vi "Stop Motor.vi"(9 "Current voltage":dbl, 10 "Desired voltage":dbl, 11 "Refnum in":refnum<k21>) -> ()   [LabVIEW 2018]
uses:
  <vilib>/Analysis/NI_AALBase.lvlib
  <vilib>/Analysis/1siggen.llb/Ramp Pattern by Samples.vi
  Samples per channle (Generation) - Global Variable.vi
  <vilib>/DAQmx/write.llb/DAQmx Write (Analog 1D DBL 1Chan NSamp).vi
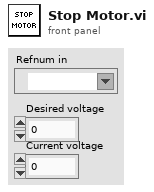
[diagram p1: front panel]
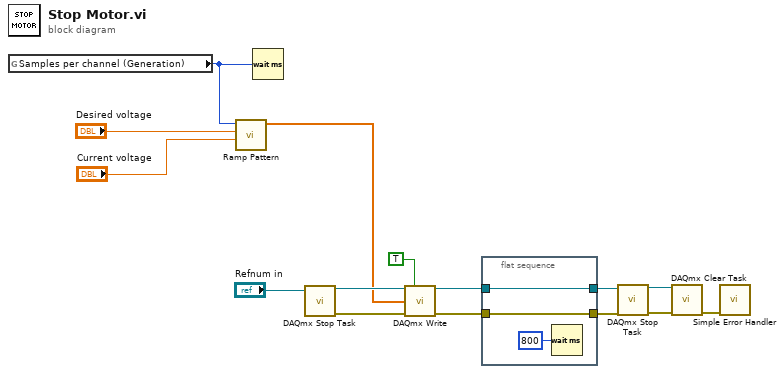
[diagram p0: block diagram]
diagram:
  n1 = global read "Samples per channle (Generation) - Global Variable.vi" "Samples per channel (Generation)"() -> (w8:i32)
  n2 = call-poly <vilib>:"Ramp Pattern.vi"("start"="Current voltage", "end"="Desired voltage", "samples"=w8) -> ("Ramp Pattern"=w9:dbl[])  [unwired: 7 in, 1 out]
  n3 = Wait (ms)(milliseconds to wait=w8) -> ()  [unwired: 1 out]
  n4 = call <vilib>:"DAQmx Stop Task.vi"("task/channels in"="Refnum in") -> ("task out"=w12:refnum<k21>, "error out"=w13:errorcluster)  [unwired: 13 in]
  n5 = call-poly <vilib>:"DAQmx Write.vi"("task/channels in"=w12, "auto start"=TRUE, "data"=w9, "error in"=w13) -> ("task out"=w4:refnum<k21>, "error out"=w2:errorcluster)  [unwired: 9 in, 1 out]
  n6 = flat-sequence {
    tunnel: w4 -> [w18]
    tunnel: [w18] -> w3
    tunnel: w2 -> [w17]
    tunnel: [w17] -> w1
    frame #0 {
      n7 = Wait (ms)(milliseconds to wait=u32 800) -> ()  [unwired: 1 out]
    }
  }
  n8 = call <vilib>:"DAQmx Stop Task.vi"("task/channels in"=w3, "error in"=w1) -> ("task out"=w5:refnum<k21>, "error out"=w6:errorcluster)  [unwired: 12 in]
  n9 = call <vilib>:"DAQmx Clear Task.vi"("task in"=w5, "error in"=w6) -> ("error out"=w7:errorcluster)  [unwired: 13 in]
  n10 = call <vilib>:"Simple Error Handler.vi"("error in (no error)"=w7) -> ()  [unwired: 4 in, 5 out]
